vi "Serial_Send.vi"(8 "error in":errorcluster, 9 "data":u8[](array[numeric]), 10 "messageID":u32, 11 "VISA resource name":refnum<visa-resource-name>) -> (0 "error out":errorcluster, 3 "VISA resource name out":refnum<visa-resource-name>)   [LabVIEW 2009, in "Serial.lvlib"]
doc: "Sends message to the serial port. To be used instead of CAN Send VI from CAN for Jaguar FRC library"
uses:
  Serial.lvlib
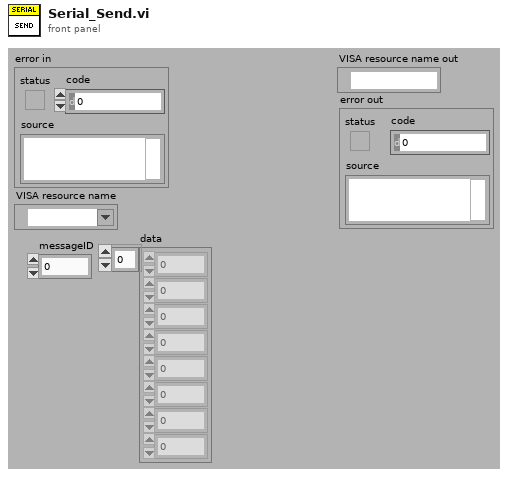
[diagram p1: front panel]
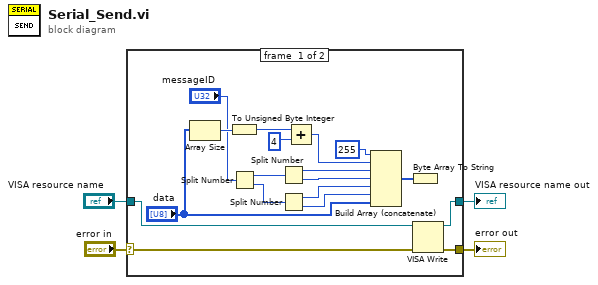
[diagram p0: block diagram]
diagram:
  n1 = case shown="No Error" "error in" {
    selector: "error in" -> [w20 w24]
    tunnel: [w21 w24] -> w3
    tunnel: "VISA resource name" -> [w19 w23]
    tunnel: [w22 w23] -> w1
    frame #0 {
      n2 = Array Size(array="data") -> (size(s)=w11:i32)
      n3 = To Unsigned Byte Integer(number=w11) -> (unsigned 8bit integer=w12:u8)
      n4 = Split Number(x="messageID") -> (hi(x)=w6:u16, lo(x)=w7:u16)
      n5 = Split Number(x=w6) -> (hi(x)=w13:u8, lo(x)=w14:u8)
      n6 = Split Number(x=w7) -> (hi(x)=w15:u8, lo(x)=w16:u8)
      n7 = Add(x=w12, y=u8 4) -> (x+y=w9:u8)
      n8 = Build Array (concatenate)(u8 255 ("element"), w9, w13, w14, w15, w16, "data") -> (w18:u8[])
      n9 = Byte Array To String(unsigned byte array=w18) -> ()  [unwired: 1 out]
      n10 = VISA Write(VISA resource name=w19, error in (no error)=w20) -> (VISA resource name out=w22:refnum<visa-resource-name>, error out=w21:errorcluster)  [unwired: 1 in, 1 out]
    }
    frame #1 {
    }
  }
  "VISA resource name out" <- w1
  "error out" <- w3
